vi "Faraday Cup Status Change.vi"(8 "error in (no error)":errorcluster, 10 "ControlQueue":refnum<queue>, 11 "DAQmxTaskContainer in":refnum<class "DAQmxTaskContainer.lvclass">) -> (0 "error out":errorcluster, 3 "DAQmxTaskContainer out":refnum<class "DAQmxTaskContainer.lvclass">)   [LabVIEW 2015, in "DAQmxTaskContainer.lvclass"]
uses:
  DAQmxTaskContainer.lvclass
  DAQmxTaskContainer.lvclass/DAQmxTaskContainer.ctl
  dependecies/ControlsVIs/Clusters-def/ProtypeCommand-DAQmxReply.ctl
  dependecies/ControlsVIs/Clusters-def/SERVER-Commands.ctl
  dependecies/ControlsVIs/Clusters-def/Standard Command.ctl
  dependecies/ControlsVIs/Clusters-def/Message types.ctl
  DAQmxTask.lvclass
  Control/Control-Server/Control-Server.lvclass
  Message/Message.lvclass
  GeneralFunctionality/GeneralFunctionality.lvclass
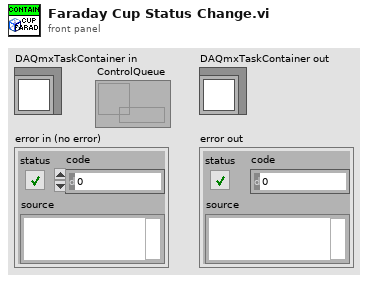
[diagram p1: front panel]
types:
  T1 = typedef "Message types.ctl" = string
  T2 = typedef "Standard Command.ctl" = cluster{"command":string, "data":variant}
  T3 = typedef "Control-Server.lvclass/SERVER-Commands.ctl" = string
  T4 = typedef "ProtypeCommand-DAQmxReply.ctl" = cluster{"On/Off":bool, "error out":errorcluster}
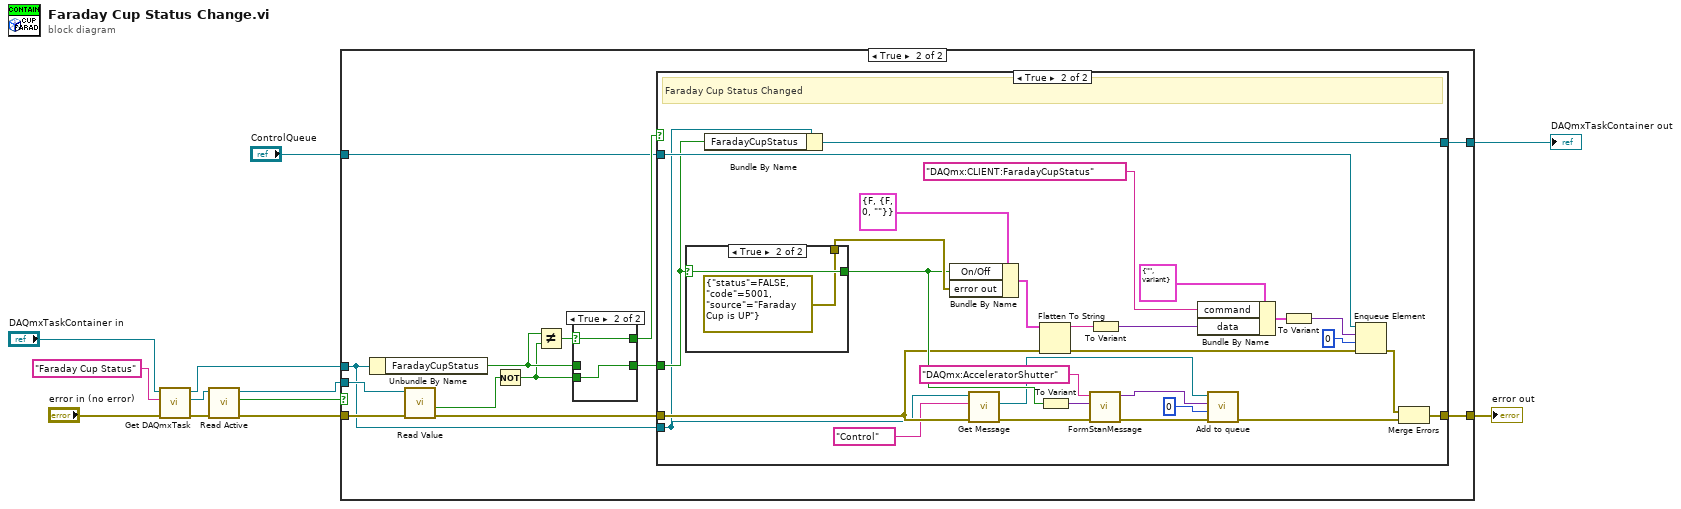
[diagram p0: block diagram]
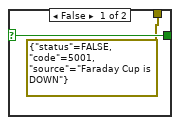
[diagram p4: hidden frame]
diagram:
  n1 = call "Get DAQmxTask.vi"("error in (no error)"="error in (no error)", "Task name"="Faraday Cup Status", "DAQmxTaskContainer in"="DAQmxTaskContainer in") -> ("error out"=w5:errorcluster, "DAQmx Task"=w7:refnum<class "DAQmxTask.lvclass">, "DAQmxTaskContainer out"=w10:refnum<class "DAQmxTaskContainer.lvclass">)  [unwired: 6 in]
  n2 = call-dynamic "Read Active.vi"("error in (no error)"=w5, "DAQmxTask in"=w7) -> ("error out"=w8:errorcluster, "Active?"=w6:bool, "DAQmxTask out"=w9:refnum<class "DAQmxTask.lvclass">)  [unwired: 7 in]
  n3 = case shown="True" w6 {
    tunnel: w8 -> [w14 w26]
    tunnel: w9 -> [_ w27]
    tunnel: w10 -> [w13 w20]
    tunnel: [w14 w18] -> w12
    tunnel: [w13 w17] -> w11
    tunnel: "ControlQueue" -> [_ w16]
    frame False {
    }
    frame True {
      n4 = Unbundle By Name(w20) -> ("FaradayCupStatus"=w24:bool)
      n5 = call-dynamic "Read Value.vi"("error in (no error)"=w26, "DAQmxTask en entrée"=w27) -> ("error out"=w19:errorcluster, "Data"=w23:bool)  [unwired: 6 in, 2 out]
      n6 = Not(x=w23) -> (.not. x?=w15:bool)
      n7 = Not Equal?(x=w24, y=w15) -> (x != y?=w25:bool)
      n8 = case shown="True" w25 {
        selector: w25 -> [w62 w64]
        tunnel: [w63 w65] -> w21
        tunnel: w24 -> [w63 _]
        tunnel: w15 -> [_ w65]
        tunnel: [w62 w64] -> w22
        frame False {
        }
        frame True {
        }
      }
      n9 = case shown="True" w22 {
        tunnel: [w29 w48] -> w17
        tunnel: w21 -> [_ w42]
        tunnel: w20 -> [w29 w31]
        tunnel: w19 -> [w28 w33]
        tunnel: [w28 w44] -> w18
        tunnel: w16 -> [_ w43]
        frame False {
        }
        frame True {
          # "Faraday Cup Status Changed"
          n10 = case shown="True" w42 {
            selector: w42 -> [w59 w61]
            tunnel: [w59 w61] -> w34
            tunnel: [errorcluster {"status"=FALSE, "code"=5001, "source"="Faraday Cup is DOWN"} ("error out") errorcluster {"status"=FALSE, "code"=5001, "source"="Faraday Cup is UP"} ("error out")] -> w52
            frame False {
            }
            frame True {
            }
          }
          n11 = Bundle By Name(cluster=w31, "FaradayCupStatus"=w42) -> (w48:refnum<class "DAQmxTaskContainer.lvclass">)
          n12 = Bundle By Name(cluster=T4 {"On/Off"=FALSE, "error out"={"status"=FALSE, "code"=0, "source"=""}} ("output cluster"), "On/Off"=w34, "error out"=w52) -> (w56:T4)
          n13 = call "Get Message.vi"("error in (no error)"=w33, "Message type"=T1 "Control", "GeneralFunctionality en entrée"=w31) -> ("error out"=w41:errorcluster, "Message.lvclass"=w30:refnum<class "Message.lvclass">)  [unwired: 6 in, 1 out]
          n14 = Flatten To String(anything=w56, error in (no error)=w33) -> (data string=w54:string, error out=w51:errorcluster)  [unwired: 2 in, 1 out]
          n15 = To Variant(anything=w34) -> (Variant=w36:variant)
          n16 = call "FormStanMessage.vi"("error in"=w41, "data"=w36, "Command"="DAQmx:AcceleratorShutter") -> ("error out"=w40:errorcluster, "message"=w39:variant)  [unwired: 7 in]
          n17 = To Variant(anything=w54) -> (Variant=w55:variant)
          n18 = Bundle By Name(cluster=T2 {"command"="", "data"=variant} ("input cluster"), "command"=T3 "DAQmx:CLIENT:FaradayCupStatus" ("Commands"), "data"=w55) -> (w50:T2)
          n19 = call "Add to queue.vi"("error in (no error)"=w40, "timeout in ms (-1)"=0, "Data"=w39, "Message in"=w30) -> ("error out"=w35:errorcluster)  [unwired: 6 in, 1 out]
          n20 = To Variant(anything=w50) -> (Variant=w49:variant)
          n21 = Enqueue Element(queue=w43, element=w49, timeout in ms (-1)=0 ("timeout en ms (-1)"), error in (no error)=w51) -> (error out=w45:errorcluster)  [unwired: 2 out]
          n22 = Merge Errors(w45, w35) -> (w44:errorcluster)
        }
      }
    }
  }
  "error out" <- w12
  "DAQmxTaskContainer out" <- w11
